vi "AI Manager Module.vi"(4 "Width goal in":u16, 6 "Bounds in":T1, 9 "Movables Channel in":T2, 10 "Communication in":refnum<class "Communication.lvclass">, 11 "Game Settings in":T3 {"FPS" items=["120"=8, "60"=16]; "Difficulty" items=["Hard"=1.0, "Medium"=0.9, "Easy"=0.8]; "Players Number" items=["2"=2, "4"=4]}) -> (0 "error out":errorcluster)   [LabVIEW 2024, in "AI Manager.lvclass"]
uses:
  AI Manager.lvclass
  Type Def/Game Settings.ctl
  Type Def/Control Device.ctl
  Type Def/Players Number.ctl
  Type Def/Difficulty.ctl
  Type Def/FPS.ctl
  Type Def/Mode.ctl
  Communication/Communication.lvclass
  <extravilib>/ChannelInstances/Tag-a[.](class'Movable')/))Channel.ctl
  Game Componants/Game Board Component/Movable/Movable.lvclass
  <vilib>/Utility/miscctls.llb/LVBoundsTypeDef.ctl
  <extravilib>/ChannelInstances/Tag-a[.](class'Movable')/Read With Abort.vi
  <extravilib>/ChannelInstances/Tag-a[.](class'Movable')/EndpointRead.vi
  <extravilib>/ChannelInstances/Tag-a[.](class'Movable').lvlib
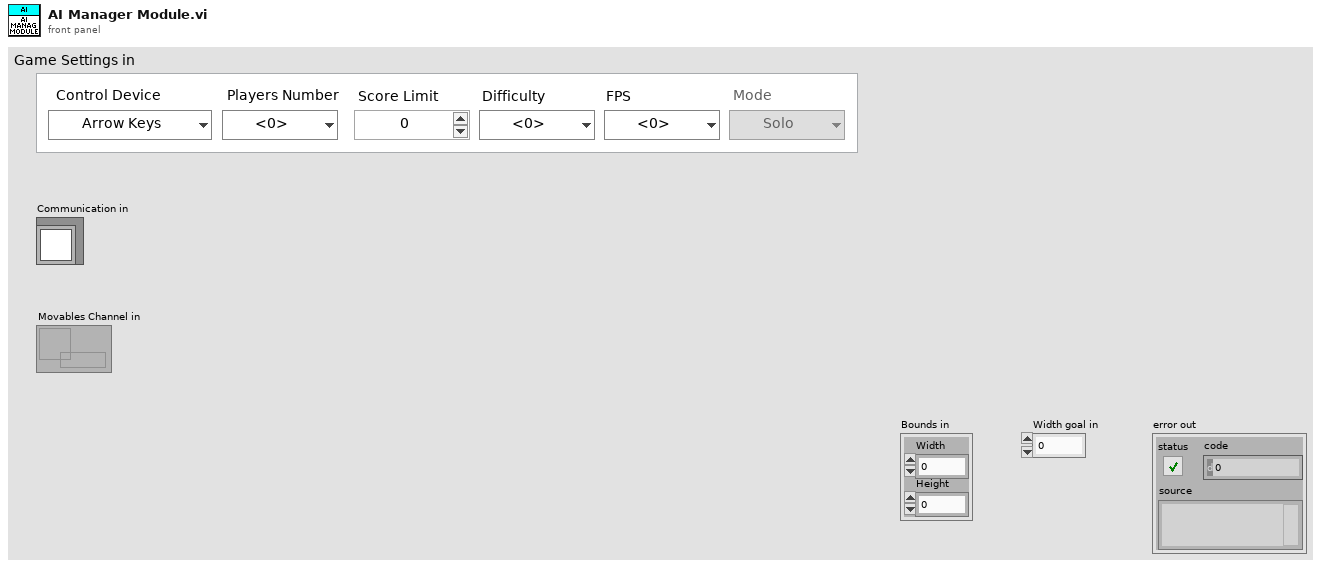
[diagram p1: front panel]
types:
  T1 = typedef "LVBoundsTypeDef.ctl" = cluster{"Width":u32, "Height":u32}
  T2 = typedef "Tag-a[.](class'Movable').lvlib/))Channel.ctl" = refnum<queue>
  T3 = typedef "Game Settings.ctl" = cluster{"Control Device":T4, "Players Number":T5, "Score Limit":u8, "Difficulty":T6, "FPS":T7, "Mode":T8, "Player ID":u8}
  T4 = typedef "Control Device.ctl" = enum16{"Arrow Keys", "Mouse", "Xbox Controller"}
  T5 = typedef "Players Number.ctl" = u16
  T6 = typedef "Difficulty.ctl" = dbl
  T7 = typedef "FPS.ctl" = u8
  T8 = typedef "Mode.ctl" = enum16{"Solo", "Multiplayer"}
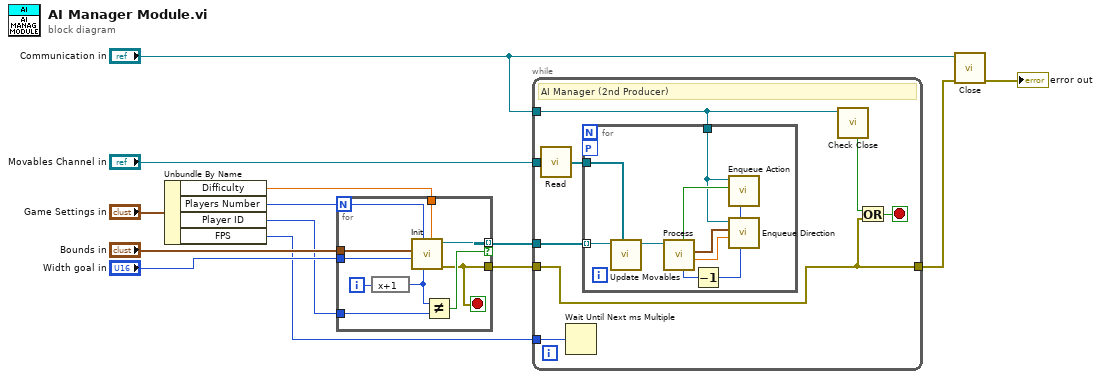
[diagram p0: block diagram]
diagram:
  n1 = Unbundle By Name("Game Settings in") -> ("Difficulty"=w12:T6, "Players Number"=w13:T5, "Player ID"=w1:u8, "FPS"=w2:T7)
  n2 = for {
    N: w13 -> [w16]
    tunnel: [w23] -> w5 mode=indexing if=w17
    tunnel: "Width goal in" -> [w22]
    tunnel: "Bounds in" -> [w21]
    tunnel: w1 -> [w18]
    tunnel: w12 -> [w15]
    tunnel: [w14] -> w6
    i -> [w20]
    stop <- w14 stop-if-true
    n3 = expression code="x+1"(w20) -> (w19:i32)
    n4 = call "Init.vi"("Difficulty"=w15, "Self Index in"=w19, "Players number in"=w16, "Right width goal in"=w22, "Bounds in"=w21) -> ("error out"=w14:errorcluster, "AI Manager out"=w23:refnum<class "AI Manager.lvclass">)  [unwired: 5 in]
    n5 = Not Equal?(x=w19, y=w18) -> (x != y?=w17:bool)
  }
  n6 = while {
    tunnel: "Communication in" -> [w24]
    tunnel: w5 -> [w31]
    tunnel: w2 -> [w30]
    tunnel: "Movables Channel in" -> [w29]
    tunnel: w6 -> [w25]
    tunnel: [w25] -> w7
    stop <- w26 stop-if-true
    # "AI Manager (2nd Producer)"
    n7 = call <extravilib>:"Read.vi"("channel"=w29) -> ("element"=w28:refnum<class "Movable.lvclass">[])  [unwired: 1 in, 1 out]
    n8 = Wait Until Next ms Multiple(millisecond multiple=w30) -> ()  [unwired: 1 out]
    n9 = for {
      tunnel: w31 -> [w40] mode=indexing
      tunnel: w28 -> [w38]
      workers-P: _ -> [_]
      tunnel: w24 -> [w35]
      n10 = call "Update Movables.vi"("Movables in"=w38, "AI Manager in"=w40) -> ("AI Manager out"=w39:refnum<class "AI Manager.lvclass">)  [unwired: 9 in]
      n11 = call "Process.vi"("AI Manager in"=w39) -> ("Velocity out"=w34:dbl, "Direction out"=w36:cluster{dbl, dbl}, "Self Index out"=w33:i32, "Boost ?"=w37:bool)  [unwired: 7 in]
      n12 = Decrement(x=w33) -> (x-1=w32:i32)
      n13 = call "Enqueue Action.vi"("Index in"=w32, "Boost in"=w37, "Communication in"=w35) -> ()  [unwired: 9 in]
      n14 = call "Enqueue Direction.vi"("Index in"=w32, "Velocity in"=w34, "Direction in"=w36, "Communication in"=w35) -> ()  [unwired: 8 in]
    }
    n15 = call "Check Close.vi"("Communication in"=w24) -> ("Stop?"=w27:bool)  [unwired: 10 in]
    n16 = Or(x=w27, y=w25) -> (x .or. y?=w26:bool)
  }
  n17 = call "Close.vi"("error in (no error)"=w7, "Communication in"="Communication in") -> ("error out"=→"error out":errorcluster)  [unwired: 9 in]
